vi "GDSControl_Disable.vi"(5 "Controls":refnum<vi>[](array[refnum]), 7 "ControlRefnum(IgnoreIfNotWired)":refnum<vi>, 11 "Disasble(True)":bool=TRUE) -> (3 "Enable Property":T1(ring))   [LabVIEW 2020]
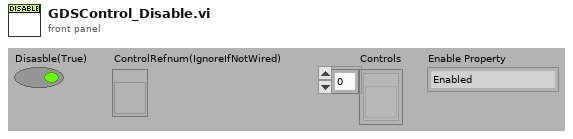
[diagram p1: front panel]
types:
  T1 = enum8{"Enabled", "Disabled", "Disabled and Grayed Out"}
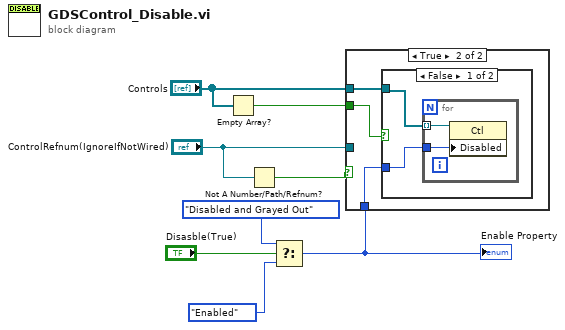
[diagram p0: block diagram]
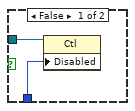
[diagram p2: hidden frame]
diagram:
  n1 = Empty Array?(array="Controls") -> (empty?=w2:bool)
  n2 = Not A Number/Path/Refnum?(number/path/refnum="ControlRefnum(IgnoreIfNotWired)") -> (NaN/Path/Refnum?=w7:bool)
  n3 = Select(t=T1."Disabled and Grayed Out" ("Enable Property"), s="Disasble(True)", f=T1."Enabled" ("Enable Property")) -> (s? t:f=w5:T1)
  "Enable Property" <- w5
  n4 = case shown="True" w7 {
    tunnel: "ControlRefnum(IgnoreIfNotWired)" -> [w10 _]
    tunnel: w5 -> [w9 w13]
    tunnel: w2 -> [_ w12]
    tunnel: "Controls" -> [_ w11]
    frame False {
      n5 = property class="Ctl"(reference=w10, "Disabled"=w9) -> ()  [unwired: 1 in, 2 out]
    }
    frame True {
      n6 = case shown="False" w12 {
        tunnel: w13 -> [w15 _]
        tunnel: w11 -> [w14 _]
        frame False {
          n7 = for {
            tunnel: w15 -> [w17]
            tunnel: w14 -> [w16] mode=indexing
            n8 = property class="Ctl"(reference=w16, "Disabled"=w17) -> ()  [unwired: 1 in, 2 out]
          }
        }
        frame True {
        }
      }
    }
  }
